vi "subParseCommandLineArgument.vi"(11 "Command line args":string[](array[string])) -> (0 "error out":errorcluster, 3 "Parameters":map{string, string}(c390))   [LabVIEW 2020, in "CommonHelpers.lvlib"]
uses:
  CommonHelpers.lvlib
  <vilib>/Utility/error.llb/whitespace.ctl
  c945251b-f142-4d30-924b-8799c887b110.vi
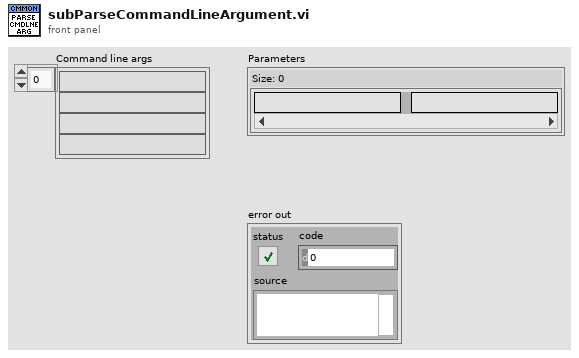
[diagram p1: front panel]
types:
  T1 = typedef "whitespace.ctl" = u16
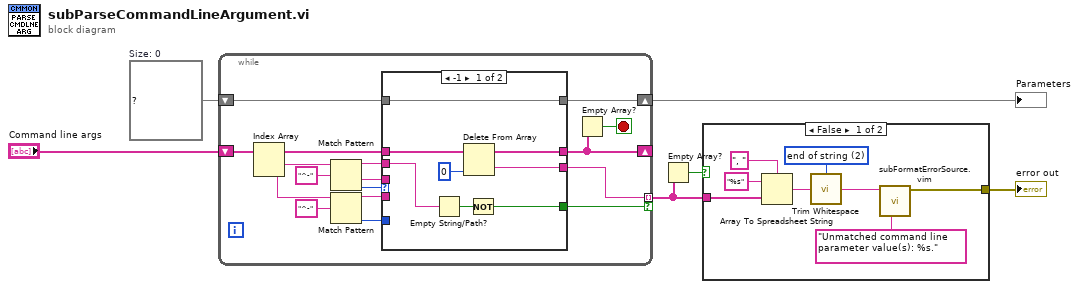
[diagram p0: block diagram]
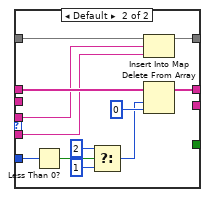
[diagram p3: hidden frame]
diagram:
  w5 = map{string, string} {}  # Size: 0
  n1 = while {
    shift-right: [w11] -> _
    shift-left: "Command line args" -> [w14]
    shift-right: [w12] -> w4
    shift-left: w5 -> [w13]
    tunnel: [w9] -> w2 mode=indexing if=w8
    stop <- w10 stop-if-true
    n2 = Index Array(array=w14) -> (element #1=w22:string, element #2=w19:string)  [unwired: 2 in]
    n3 = Match Pattern(string=w22, regular expression="^-") -> (before substring=w7:string, after substring=w17:string, offset past match=w18:i32)  [unwired: 1 in, 1 out]
    n4 = Match Pattern(string=w19, regular expression="^-") -> (before substring=w16:string, offset past match=w15:i32)  [unwired: 1 in, 2 out]
    n5 = case shown="-1" w18 {
      tunnel: w17 -> [_ w32]
      tunnel: w16 -> [_ w31]
      tunnel: w15 -> [_ w42]
      tunnel: w14 -> [w29 w40]
      tunnel: [w28 w35] -> w11
      tunnel: w13 -> [w27 w34]
      tunnel: [w27 w33] -> w12
      tunnel: [w26 _] -> w9
      tunnel: [w23 _] -> w8
      tunnel: w7 -> [w25 _]
      frame -1 {
        n6 = Empty String/Path?(string/path=w25) -> (empty?=w24:bool)
        n7 = Delete From Array(array=w29, index=0) -> (deleted portion=w26:string, array with subset deleted=w28:string[])  [unwired: 1 in]
        n8 = Not(x=w24) -> (.not. x?=w23:bool)
      }
      frame Default {
        n9 = Less Than 0?(x=w42) -> (x < 0?=w41:bool)
        n10 = Select(t=2 ("length"), s=w41, f=1 ("length")) -> (s? t:f=w36:i32)
        n11 = Insert Into Map(map in=w34, key=w32, value=w31) -> (map out=w33:map{string, string})  [unwired: 2 out]
        n12 = Delete From Array(array=w40, length=w36, index=0) -> (array with subset deleted=w35:string[])  [unwired: 1 out]
      }
    }
    n13 = Empty Array?(array=w11) -> (empty?=w10:bool)
  }
  "Parameters" <- w4
  n14 = Empty Array?(array=w2) -> (empty?=w1:bool)
  n15 = case shown="False" w1 {
    tunnel: w2 -> [w48 _]
    tunnel: [w45 _] -> w3
    frame False {
      w43 = T1 2 items=["both", "start of string", "end of string"] ("location (both)")
      n16 = Array To Spreadsheet String(delimiter (Tab)=", " ("format string"), array=w48, 3:"%s" ("format string")) -> (spreadsheet string=w47:string)
      n17 = call <vilib>:"Trim Whitespace.vi"("string"=w47, "location (both)"=w43) -> ("trimmed string"=w44:string)
      n18 = call "subFormatErrorSource.vim"("format string"="Unmatched command line parameter value(s): %s.", "Parameter cluster"=w44) -> ("Error out"=w45:errorcluster)  [unwired: 9 in]
    }
    frame True {
    }
  }
  "error out" <- w3
